vi "Comparator.vi"(5 "Previous Scan Value":dbl, 6 "Present scan array":dbl[](array[numeric]), 8 "Ch Description":T1 {"Duty" format="%016b"; "D" format="%#_5g"; "C" format="%#_5g"; "B" format="%#_5g"; "A" format="%#_5g"}, 9 "Ch names":string[](array[string])) -> (0 "String":string, 1 "Value":dbl, 3 "HelpText":string="\"A\" Warn if above this value\n\"B\" Warn if below this value\n\"C\" Hysteresis margin\n\"D\" is the averaging time in minutes\n\nWrite Channel name to check in the box above \"Comparator\"")   [LabVIEW 2016]
uses:
  ADAM Client/Sub VIs/ADAM Controls/Ch_description_ADAM.ctl
  ADAM Client/Sub VIs/ADAM Controls/Module_type_ADAM.ctl
  ADAM Client/Sub VIs/ADAM Controls/Function_ADAM.ctl
  ADAM Client/Sub VIs/ADAM Controls/Channel_State.ctl
  ADAM Client/Sub VIs/ADAM Controls/Calib_type_ADAM.ctl
  ADAM Client/Sub VIs/ADAM Controls/Address.ctl
  ADAM Client/Sub VIs/ADAM Controls/Search_mode.ctl
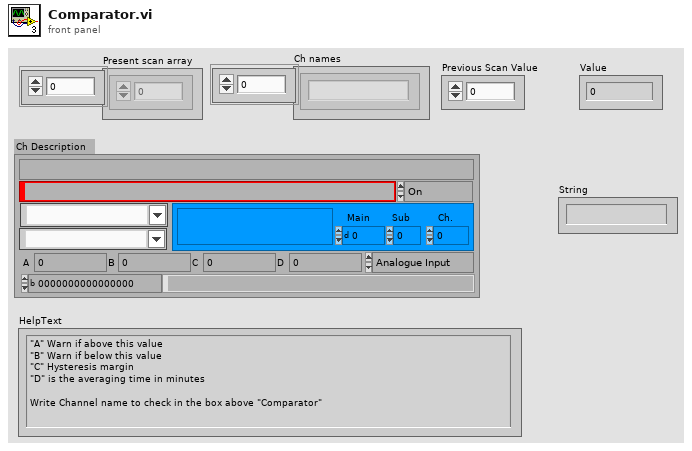
[diagram p1: front panel]
types:
  T1 = typedef "Ch_description_ADAM.ctl" = cluster{"Ch Name":string, "Type":T2, "Function":T3, "Ch State":T4, "Calibration type":T5, "A":dbl, "B":dbl, "C":dbl, "D":dbl, "Comments":string, "Address":T6, "String":string, "Duty":u16}
  T2 = typedef "Module_type_ADAM.ctl" = string
  T3 = typedef "Function_ADAM.ctl" = enum16{"Analogue Input", "Digital Input", "Event counter", "Event rate", "Analogue Output", "Digital Output", "Relay Output"}
  T4 = typedef "Channel_State.ctl" = enum16{"On", "Off", "Always On", "Always Off"}
  T5 = typedef "Calib_type_ADAM.ctl" = string
  T6 = typedef "Address.ctl" = cluster{"Main":i32, "Ch.":i32, "Sub":i32, "Port Name":string}
  T7 = typedef "Search_mode.ctl" = enum16{"Between times", "All Times"}
  T8 = cluster{"Centre Times":dbl[], "Output array":dbl[]}
  T9 = cluster{"Centre Times":dbl[], "Output array":dbl[]}[]
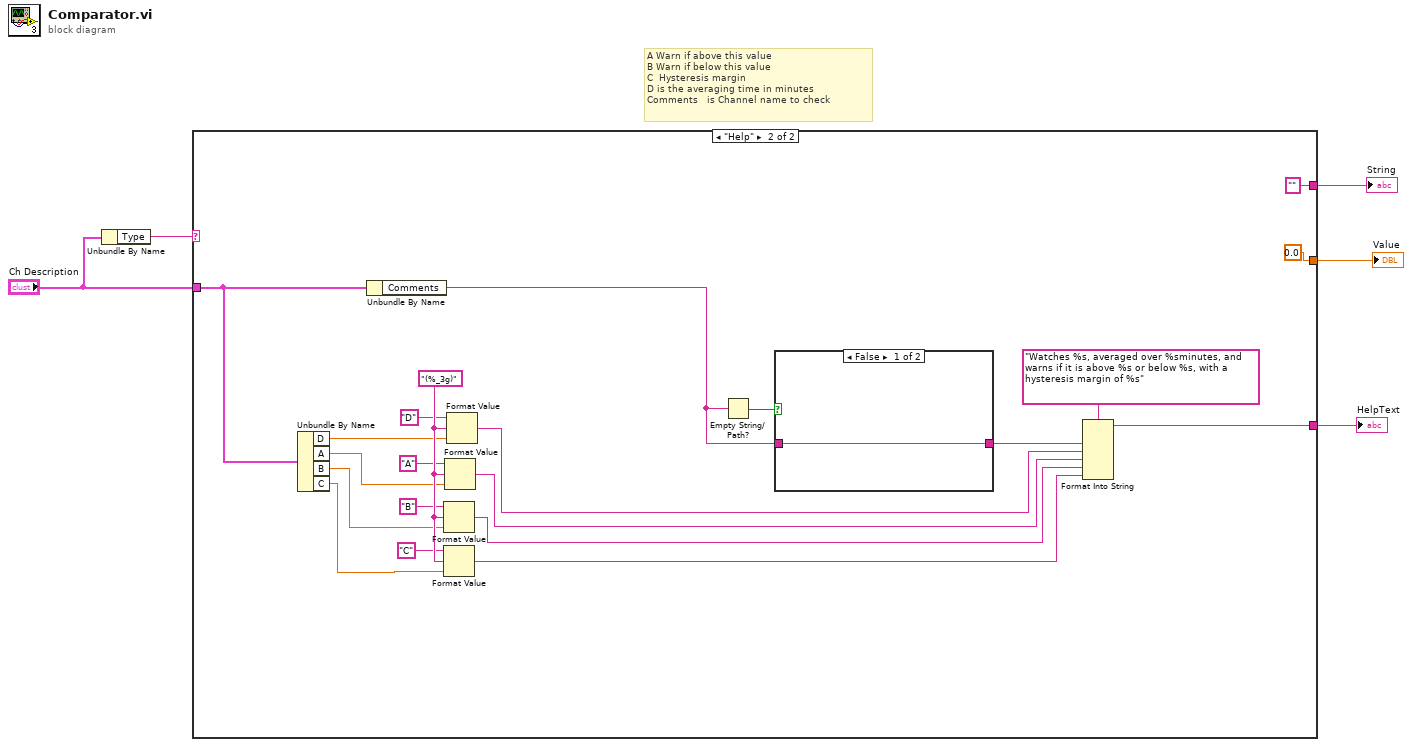
[diagram p0: block diagram]
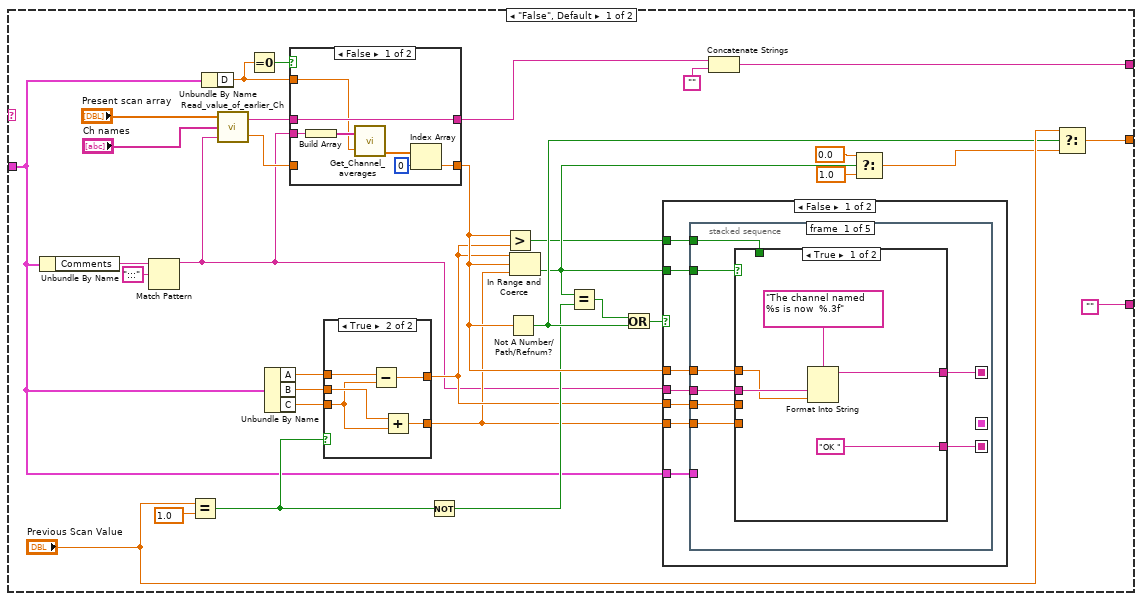
[diagram p2: hidden frame]
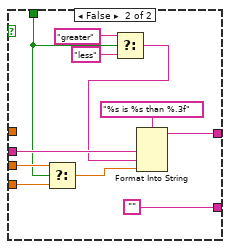
[diagram p5: hidden frame]
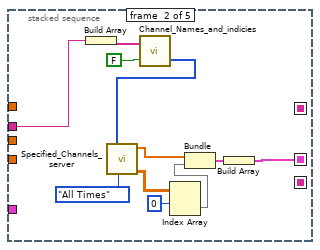
[diagram p6: hidden frame]
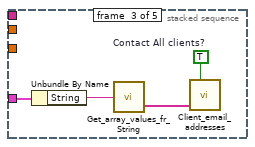
[diagram p7: hidden frame]
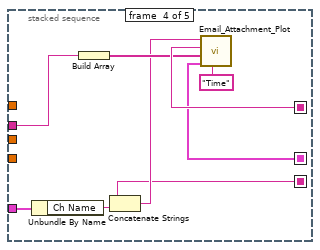
[diagram p8: hidden frame]
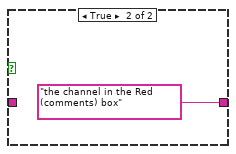
[diagram p11: hidden frame]
diagram:
  # "A Warn if above this value\nB Warn if below this value\nC  Hysteresis margin\nD is the averaging time in minutes\nComments   is Channel name to check"
  n1 = Unbundle By Name("Ch Description") -> ("Type"=w2:T2)
  n2 = case shown="\"Help\"" w2 {
    tunnel: [w37 0.0 ("f")] -> w5
    tunnel: [w16 ""] -> w4
    tunnel: "Ch Description" -> [w7 w117]
    tunnel: ["" w118] -> w1
    frame "False", Default {
      n3 = Unbundle By Name(w7) -> ("Comments"=w38:string)
      n4 = Match Pattern(string=w38, regular expression=":::" ("String to match")) -> (before substring=w13:string)  [unwired: 4 out]
      n5 = Equal?(x="Previous Scan Value", y=1.0) -> (x = y?=w20:bool)
      n6 = Unbundle By Name(w7) -> ("D"=w28:dbl)
      n7 = call "Read_value_of_earlier_Ch.vi"("Desired Ch to Read"=w13, "Ch names"="Ch names", "Present scan array"="Present scan array") -> ("Value"=w29:dbl, "Scan comment"=w15:string)  [unwired: 1 in]
      n8 = Equal To 0?(x=w28) -> (x = 0?=w30:bool)
      n9 = Unbundle By Name(w7) -> ("A"=w17:dbl, "B"=w18:dbl, "C"=w19:dbl)
      n10 = case shown="False" w30 {
        tunnel: [w50 w53] -> w9
        tunnel: w13 -> [w52 _]
        tunnel: [w48 w54] -> w31
        tunnel: w28 -> [w46 _]
        tunnel: w29 -> [_ w54]
        tunnel: w15 -> [w50 w53]
        frame False {
          n11 = Build Array(w52) -> (w47:string[])
          n12 = call "Get_Channel_averages.vi"("Desired Ch Names"=w47, "Averaging time (mins)"=w46) -> ("number"=w49:dbl[])  [unwired: 1 in, 2 out]
          n13 = Index Array(array=w49, index=0) -> (element=w48:dbl)
        }
        frame True {
        }
      }
      n14 = case shown="True" w20 {
        tunnel: [w40 w45] -> w22
        tunnel: w17 -> [w40 w44]
        tunnel: w18 -> [w39 w43]
        tunnel: [w39 w41] -> w21
        tunnel: w19 -> [_ w42]
        frame False {
        }
        frame True {
          n15 = Subtract(x=w44, y=w42) -> (x-y=w45:dbl)
          n16 = Add(x=w43, y=w42) -> (x+y=w41:dbl)
        }
      }
      n17 = Not(x=w20) -> (.not. x?=w27:bool)
      n18 = Greater?(x=w31, y=w22) -> (0:w23:bool)
      n19 = Not A Number/Path/Refnum?(number/path/refnum=w31) -> (NaN/Path/Refnum?=w34:bool)
      n20 = In Range and Coerce(upper limit=w22, x=w31, lower limit=w21) -> (In Range?=w26:bool)  [unwired: 1 out]
      n21 = Equal?(x=w26, y=w27) -> (x = y?=w32:bool)
      n22 = Or(x=w32, y=w34) -> (x .or. y?=w33:bool)
      n23 = case shown="False" w33 {
        tunnel: w13 -> [w61 _]
        tunnel: w22 -> [w60 _]
        tunnel: w7 -> [w59 _]
        tunnel: w21 -> [w58 _]
        tunnel: w26 -> [w57 _]
        tunnel: w31 -> [w56 _]
        tunnel: w23 -> [w55 _]
        frame False {
          n24 = stacked-sequence {
            seq-local: [w67 _ _ _ _] -> [_ _ _ w108 _]
            seq-local: [_ w87 _ _ _] -> [_ _ _ w105 _]
            seq-local: [w65 _ _ _ _] -> [_ _ _ w101 _]
            tunnel: w61 -> [w69 w95 _ w107 _]
            tunnel: w60 -> [w68 _ _ _ _]
            tunnel: w59 -> [_ _ w100 w109 _]
            tunnel: w58 -> [w66 _ _ _ _]
            tunnel: w57 -> [w64 _ _ _ _]
            tunnel: w56 -> [w63 _ _ _ _]
            tunnel: w55 -> [w62 _ _ _ _]
            frame #0 {
              n25 = case shown="True" w64 {
                tunnel: w69 -> [w74 w85]
                tunnel: w68 -> [_ w78]
                tunnel: [w72 w84] -> w67
                tunnel: w66 -> [_ w77]
                tunnel: ["OK " ""] -> w65
                tunnel: w63 -> [w70 _]
                tunnel: w62 -> [_ w75]
                frame True {
                  n26 = Format Into String(format string="The channel named %s is now  %.3f" ("Format String"), w74, w70) -> (resulting string=w72:string)  [unwired: 2 in, 1 out]
                }
                frame False {
                  n27 = Select(t=w78, s=w75, f=w77) -> (s? t:f=w76:dbl)
                  n28 = Select(t="greater", s=w75, f="less") -> (s? t:f=w80:string)
                  n29 = Format Into String(format string="%s is %s than %.3f" ("Format String"), w85, w80, w76) -> (resulting string=w84:string)  [unwired: 2 in, 1 out]
                }
              }
            }
            frame #1 {
              n30 = Build Array(w95) -> (w94:string[])
              n31 = call "Channel_Names_and_indicies.vi"("All Active Channels"=FALSE, "Desired Ch Names"=w94) -> ("Indicies"=w92:i32[])  [unwired: 1 out]
              n32 = call "Specified_Channels_server.vi"("Mode"=Search_mode."All Times", "Requested channels"=w92) -> ("Output array"=w90:dbl[][], "Centre Times"=w86:dbl[])  [unwired: 3 in, 3 out]
              n33 = Index Array(array=w90, index (row)=0) -> (element=w88:dbl[])  [unwired: 1 in]
              n34 = Bundle("Centre Times"=w86, "Output array"=w88) -> (w91:T8)  [unwired: 1 out]
              n35 = Build Array(w91) -> (w87:T9)
            }
            frame #2 {
              w98 = TRUE  # Contact All clients?
              n36 = Unbundle By Name(w100) -> ("String"=w99:string)
              n37 = call "Get_array_values_fr_String.vi"("String Value"=w99) -> ("String array"=w97:string[])  [unwired: 1 out]
              n38 = call "Client_email_addresses.vi"("Extra People to Email"=w97, "Contact All clients?"=w98) -> ()  [unwired: 1 in]
            }
            frame #3 {
              n39 = Unbundle By Name(w109) -> ("Ch Name"=w102:string)
              n40 = Build Array(w107) -> (w106:string[])
              n41 = Concatenate Strings(w101, w102) -> (w103:string)
              n42 = call "Email_Attachment_Plot.vi"("X axis name"="Time", "XY Graph"=w105, "Series Names"=w106, "message"=w108, "subject ([No Subject])"=w103) -> ()  [unwired: 1 in, 1 out]
            }
            frame #4 {
            }
          }
        }
        frame True {
        }
      }
      n43 = Concatenate Strings(w9, "") -> (w16:string)
      n44 = Select(t=0.0, s=w26, f=1.0) -> (s? t:f=w35:dbl)
      n45 = Select(t="Previous Scan Value", s=w34, f=w35) -> (s? t:f=w37:dbl)
    }
    frame "Help" {
      w126 = "(%_3g)" ("format string")
      n46 = Unbundle By Name(w117) -> ("D"=w121:dbl, "A"=w123:dbl, "B"=w125:dbl, "C"=w115:dbl)
      n47 = Unbundle By Name(w117) -> ("Comments"=w116:string)
      n48 = Format Value(string ("")="B", format string=w126, value (0)=w125) -> (output string=w124:string)
      n49 = Format Value(string ("")="C", format string=w126, value (0)=w115) -> (output string=w114:string)
      n50 = Format Value(string ("")="A", format string=w126, value (0)=w123) -> (output string=w122:string)
      n51 = Format Value(string ("")="D", format string=w126, value (0)=w121) -> (output string=w120:string)
      n52 = Empty String/Path?(string/path=w116) -> (empty?=w128:bool)
      n53 = case shown="False" w128 {
        tunnel: [w131 "the channel in the Red (comments) box"] -> w127
        tunnel: w116 -> [w131 _]
        frame False {
        }
        frame True {
        }
      }
      n54 = Format Into String(format string="Watches %s, averaged over %sminutes, and warns if it is above %s or below %s, with a hysteresis margin of %s", w127, w120, w122, w124, w114) -> (resulting string=w118:string)  [unwired: 2 in, 1 out]
    }
  }
  "Value" <- w5
  "String" <- w4
  "HelpText" <- w1
